vi "test Multiple Actor Core.vi"(8 "error in (no error)":errorcluster, 11 "TestCase in":refnum<class "Monitor Test.lvclass">) -> (0 "error out":errorcluster, 3 "TestCase out":refnum<class "Monitor Test.lvclass">)   [LabVIEW 2017, in "Monitor Test.lvclass"]
uses:
  Monitor Test.lvclass
  Test Actor/Test Actor.lvclass
  C:/Program Files (x86)/National Instruments/LabVIEW 2017/vi.lib/ActorFramework/Actor/Actor.lvclass
  <vilib>/ActorFramework/Message Enqueuer/Message Enqueuer.lvclass/Message Enqueuer.ctl
  <vilib>/ActorFramework/Message Enqueuer/Enqueue.vi
  <vilib>/ActorFramework/Stop Msg/Stop Msg.lvclass
  C:/Program Files (x86)/National Instruments/LabVIEW 2017/vi.lib/ActorFramework/Message/Message.lvclass
  <vilib>/ActorFramework/Message Priority Queue/Priority Enqueue.vi
  <vilib>/ActorFramework/Actor/Actor.lvclass
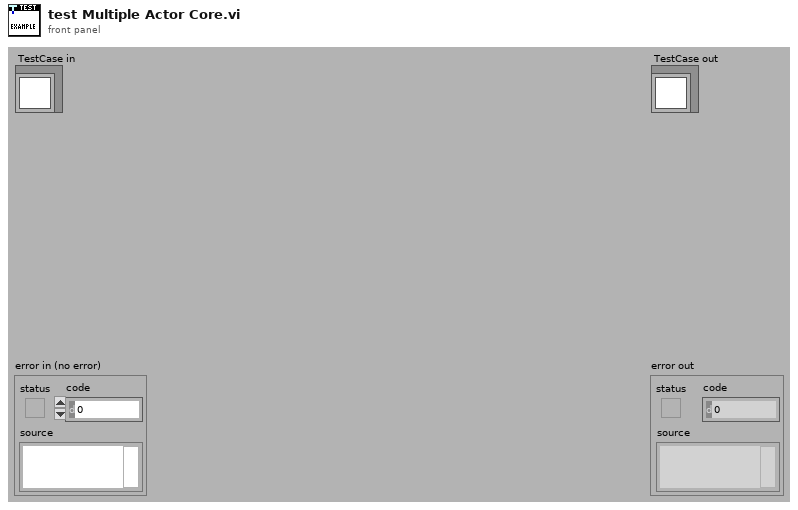
[diagram p1: front panel]
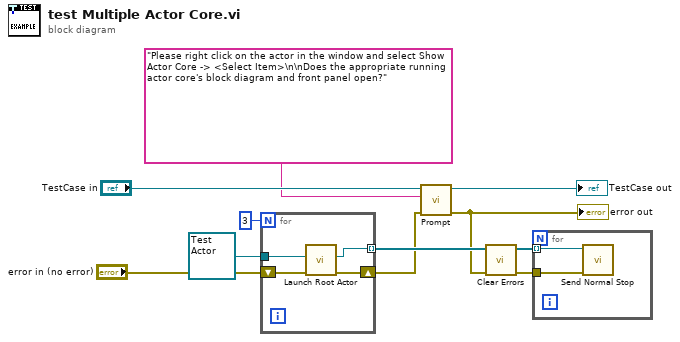
[diagram p0: block diagram]
diagram:
  n1 = for {
    N: 3 -> [_]
    tunnel: [w14] -> w10 mode=indexing
    tunnel: refnum<class "Test Actor.lvclass"> refnum ("Test Actor.lvclass") -> [w11]
    shift-right: [w12] -> w5
    shift-left: "error in (no error)" -> [w13]
    n2 = call <vilib>:"Launch Root Actor.vi"("error in (no error)"=w13, "Actor"=w11) -> ("error out"=w12:errorcluster, "Actor's Enqueuer"=w14:refnum<class "Message Enqueuer.lvclass">)  [unwired: 8 in]
  }
  n3 = call "Prompt.vi"("error in (no error)"=w5, "Prompt"="Please right click on the actor in the window and select Show Actor Core -> <Select Item>\n\nDoes the appropriate running actor core's block diagram and front panel open?", "Monitor Test in"="TestCase in") -> ("error out"=w4:errorcluster, "Monitor Test out"=→"TestCase out":refnum<class "Monitor Test.lvclass">)  [unwired: 7 in]
  "error out" <- w4
  n4 = call <vilib>:"Clear Errors.vi"("error in (no error)"=w4) -> ("error out"=w3:errorcluster)  [unwired: 5 in, 1 out]
  n5 = for {
    tunnel: w10 -> [w16] mode=indexing
    tunnel: w3 -> [w15]
    n6 = call <vilib>:"Send Normal Stop.vi"("error in (no error)"=w15, "Message Enqueuer"=w16) -> ()  [unwired: 9 in, 1 out]
  }
